vi "Calculate Makespan (Prins FIFO Engine).vi"(8 "error in (no error)":errorcluster, 9 "Reorder?":bool, 10 "Schedule In":u16[](array[numeric]), 11 "OSSP_Problem in":refnum<class "OSSP_Problem.lvclass">) -> (0 "error out":errorcluster, 1 "Makespan":i32, 2 "Schedule Out":u16[](array[numeric]), 3 "OSSP_Problem out":refnum<class "OSSP_Problem.lvclass">)   [LabVIEW 2013, in "Scheduler.lvclass"]
uses:
  Scheduler.lvclass
  OSSP_Problem.lvclass
  OSSP_Problem.lvclass/OSSP_Problem.ctl
  UpdateMachineGaps.vi
  UpdateJobGaps.vi
  Find Intersecting Gaps.vi
  Transform to Plain Job and Machine Gaps Array.vi
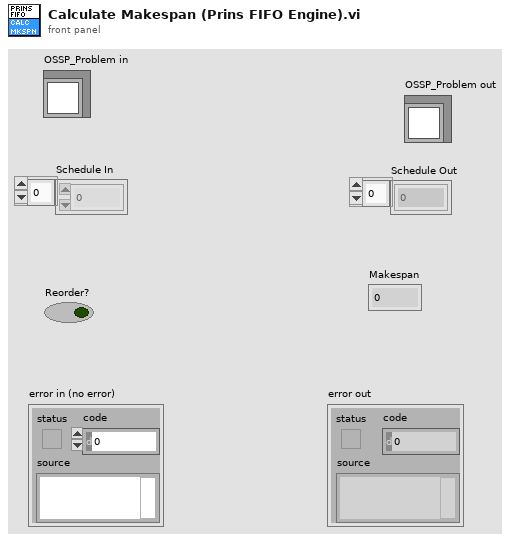
[diagram p1: front panel]
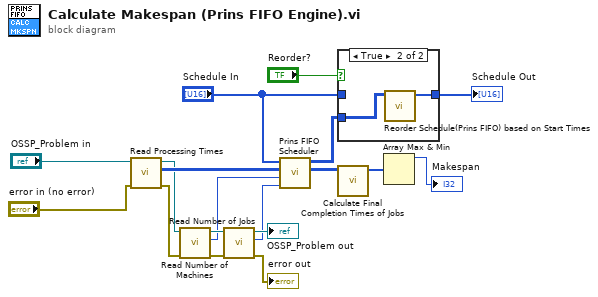
[diagram p0: block diagram]
diagram:
  n1 = call "Read Processing Times.vi"("error in (no error)"="error in (no error)", "OSSP_Problem in"="OSSP_Problem in") -> ("error out"=w1:errorcluster, "Processing Times"=w5:u16[][], "OSSP_Problem out"=w2:refnum<class "OSSP_Problem.lvclass">)  [unwired: 7 in]
  n2 = call "Read Number of Machines.vi"("error in (no error)"=w1, "OSSP_Problem in"=w2) -> ("error out"=w10:errorcluster, "Number of Machines"=w4:i32, "OSSP_Problem out"=w11:refnum<class "OSSP_Problem.lvclass">)  [unwired: 7 in]
  n3 = call "Read Number of Jobs.vi"("error in (no error)"=w10, "OSSP_Problem in"=w11) -> ("error out"=→"error out":errorcluster, "Number of Jobs"=w3:i32, "OSSP_Problem out"=→"OSSP_Problem out":refnum<class "OSSP_Problem.lvclass">)  [unwired: 7 in]
  n4 = call "Prins FIFO Scheduler.vi"("Number of Jobs"=w3, "Number of Machines"=w4, "Processing Times(MxJ)"=w5, "Schedule In"="Schedule In") -> ("Completion Times (MxJ)"=w16:i32[][], "Start Times (MxJ)"=w15:i32[][])  [unwired: 6 in]
  n5 = case shown="True" "Reorder?" {
    tunnel: [w19 w21] -> w17
    tunnel: w15 -> [_ w20]
    tunnel: "Schedule In" -> [w19 _]
    frame False {
    }
    frame True {
      n6 = call "Reorder Schedule(Prins FIFO) based on Start Times.vi"("Start Times (MxJ)"=w20) -> ("Reordered Schedule(Prins FIFO)"=w21:u16[])  [unwired: 10 in]
    }
  }
  "Schedule Out" <- w17
  n7 = call "Calculate Final Completion Times of Jobs.vi"("Completion Times (MxJ)"=w16) -> ("Job Completion Times"=w14:i32[])  [unwired: 10 in]
  n8 = Array Max & Min(array=w14) -> (max value=→"Makespan":i32)  [unwired: 3 out]
